vi "ReadCam0Attributes-LoadFile.vi"() -> ()   [LabVIEW 2017]
uses:
  <vilib>/vision/driver/IMAQdx.llb/IMAQdx Camera Control Mode.ctl
  <vilib>/vision/driver/NI_Vision_Acquisition_Software.lvlib
panel:
  out "error out":errorcluster
  in  "Camera Name":refnum<k21> caption="IMAQdx Session"
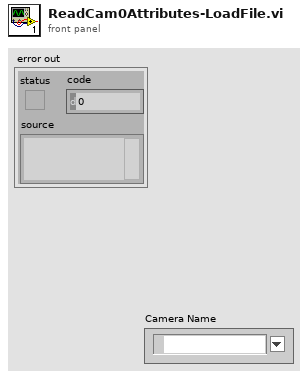
[diagram p1: front panel]
types:
  T1 = typedef "NI_Vision_Acquisition_Software.lvlib/IMAQdx Camera Control Mode.ctl" = enum32{"Controller", "Listener"}
  T2 = typedef "IMAQdx.ctl" = refnum<k21>
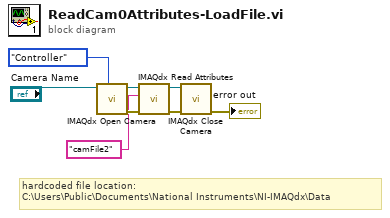
[diagram p0: block diagram]
diagram:
  # "hardcoded file location:\nC:\\Users\\Public\\Documents\\National Instruments\\NI-IMAQdx\\Data"
  n1 = call <vilib>:"IMAQdx Open Camera.vi"("Camera Control Mode"=IMAQdx_Camera_Control_Mode."Controller", "Session In"="Camera Name") -> ("error out"=w7:errorcluster, "Session Out"=w8:T2)  [unwired: 1 in, 7 out]
  n2 = call <vilib>:"IMAQdx Read Attributes.vi"("error in"=w7, "Filename"="camFile2", "Session In"=w8) -> ("error out"=w6:errorcluster, "Session Out"=w1:T2)  [unwired: 7 in]
  n3 = call <vilib>:"IMAQdx Close Camera.vi"("error in"=w6, "Session In"=w1) -> ("error out"=→"error out":errorcluster)  [unwired: 1 in, 8 out]
